vi "test-cubic-spline-02.vi"() -> (3 "Test Passed":bool)   [LabVIEW 2019]
uses:
  <vilib>/Rock Robotics/WPI/ThirdParty/JAS_Junk/TrajLib/POSEwCURVATURE.ctl
  <vilib>/Rock Robotics/WPI/ThirdParty/JAS_Junk/TrajLib/POSE2D.ctl
  <vilib>/Rock Robotics/WPI/ThirdParty/JAS_Junk/TrajLib/TRANSLATION2D.ctl
  <vilib>/Rock Robotics/WPI/ThirdParty/JAS_Junk/TrajLib/ROTATION2D.ctl
  <vilib>/Rock Robotics/WPI/ThirdParty/JAS_Junk/TrajLib/Rotation2d_CreateAngle.vi
  <vilib>/Rock Robotics/WPI/ThirdParty/JAS_Junk/TrajLib/Util_CalcDist.vi
  <vilib>/Rock Robotics/WPI/ThirdParty/JAS_Junk/TrajLib/Trajectory_Library.lvlib
panel:
  out "XY Graph":cluster{dbl[], dbl[]}(graph)
  out "All Interior \nwayPoints\nFound (True)":bool
  out "end rot = 0":dbl
  out "end y = 0":dbl
  out "end x = 0":dbl
  out "start rot = 0":dbl
  out "start y = 0":dbl
  out "start x = 0":dbl
  out "max dtheta < 0.0872":dbl
  out "max dy < 0.00127":dbl
  out "max dx  < 0.127":dbl
  out "Overall Error":errorcluster
  out "Elements":i32
  out "Create Spline Error":errorcluster
  out "SplinePoses\nWCurve":T1[](array[typedef]) {"POSE"."ROTATION"."SIN" format="%13.4f"; "POSE"."ROTATION"."COS" format="%13.4f"; "POSE"."ROTATION"."VALUE" format="%13.4f"; "POSE"."TRANSLATION"."Y" format="%14.3f"; "POSE"."TRANSLATION"."X" format="%14.3f"}
  out "Elapsed Time":dbl
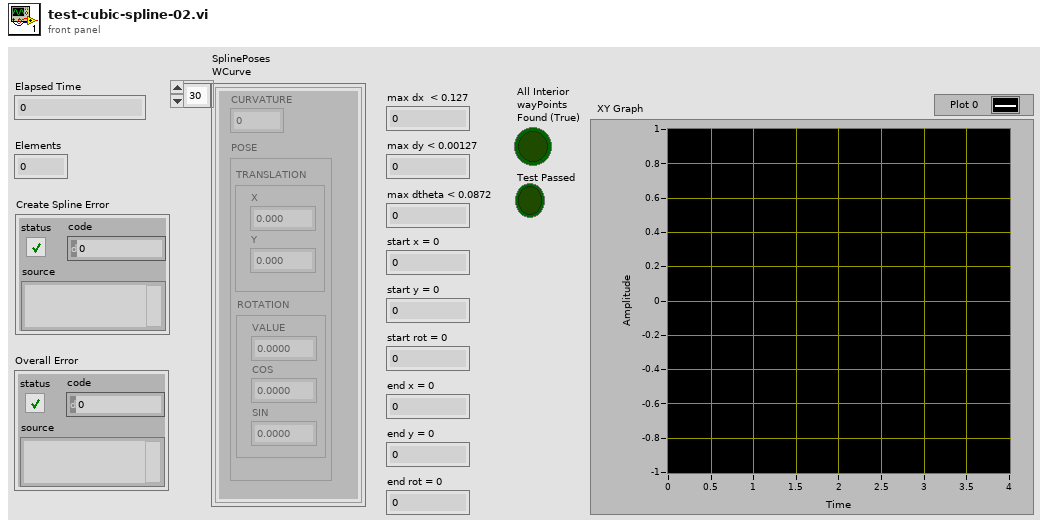
[diagram p1: front panel]
types:
  T1 = typedef "Trajectory_Library.lvlib/POSEwCURVATURE.ctl" = cluster{"CURVATURE":dbl, "POSE":T2}
  T2 = typedef "Trajectory_Library.lvlib/POSE2D.ctl" = cluster{"TRANSLATION":T3, "ROTATION":T4}
  T3 = typedef "Trajectory_Library.lvlib/TRANSLATION2D.ctl" = cluster{"X":dbl, "Y":dbl}
  T4 = typedef "Trajectory_Library.lvlib/ROTATION2D.ctl" = cluster{"VALUE":dbl, "COS":dbl, "SIN":dbl}
  T5 = typedef "Trajectory_Library.lvlib/SPLINE_CTRL_VECTOR.ctl" = cluster{"Xs":dbl[], "Ys":dbl[]}
  T6 = typedef "Trajectory_Library.lvlib/SPLINE.ctl" = cluster{"Degree":i32, "Coefficients":T7}
  T7 = typedef "NI_Matrix.lvlib/RealMatrix.ctl" = dbl[][]
  T8 = typedef "Trajectory_Library.lvlib/TWIST2D.ctl" = cluster{"dX":dbl, "dY":dbl, "dTHETA":dbl}
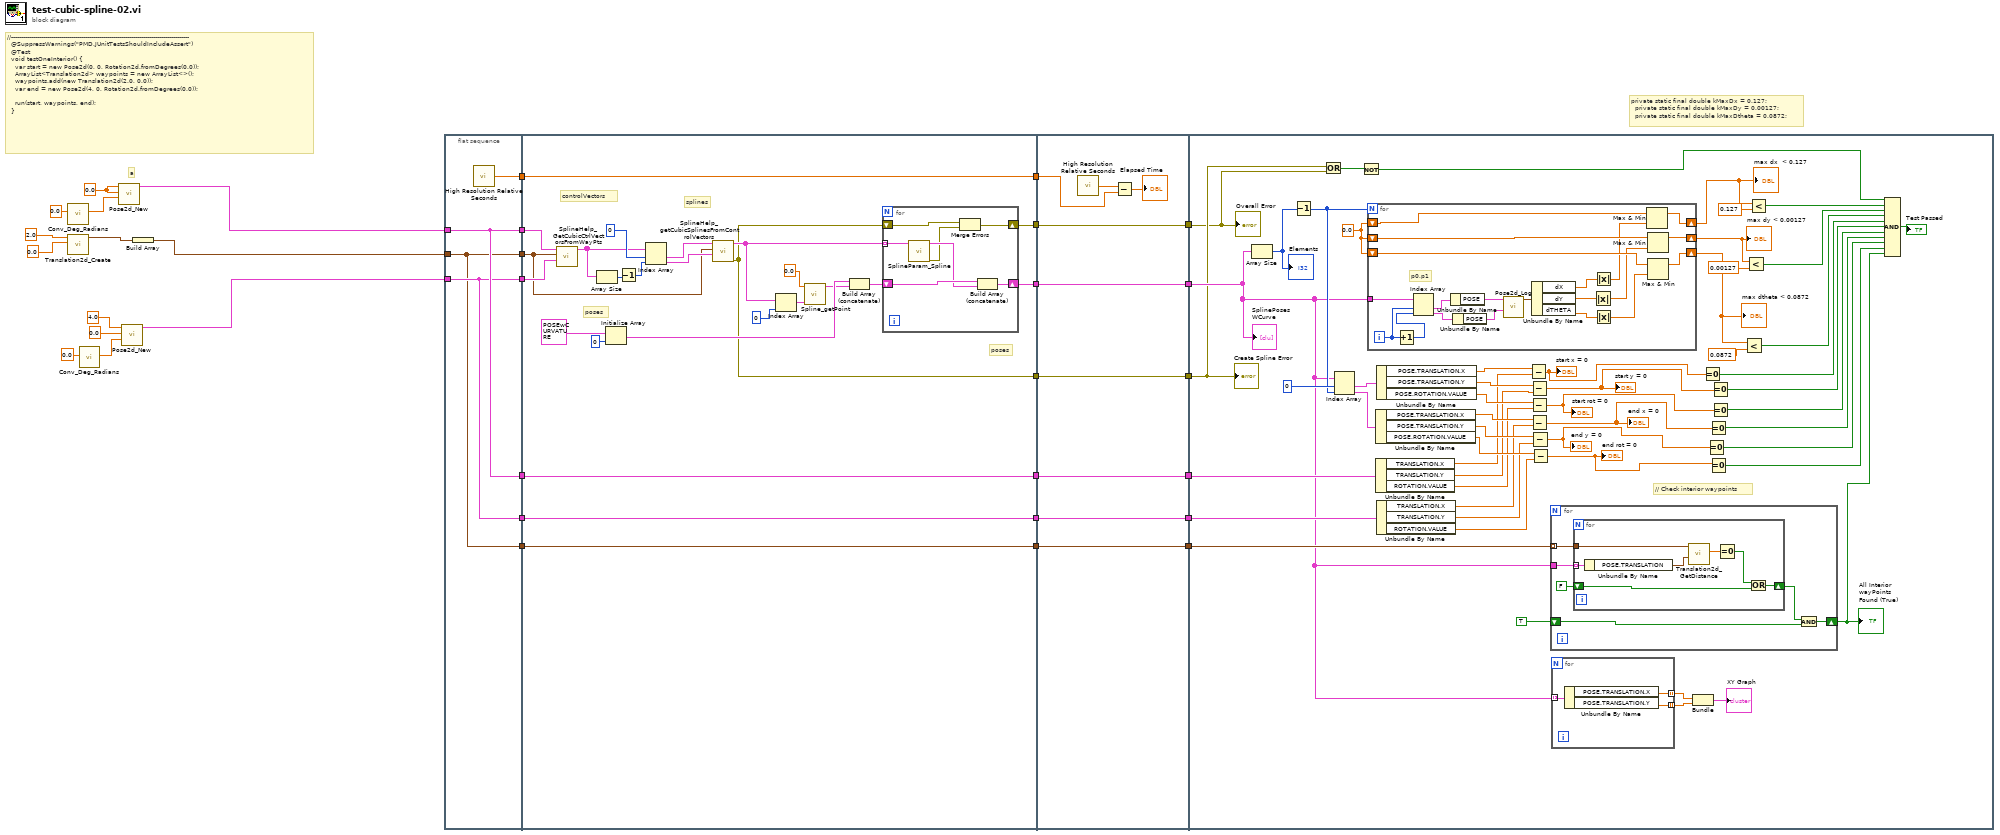
[diagram p0: block diagram]
diagram:
  w11 = 0.0 ("X")
  # "a"
  # "//-----------------------------------------------------------------------------------------\n  @SuppressWarnings(\"PMD.JUnitTestsShouldIncludeAssert\")\n  @Test\n  void testOneInterior() {\n    var start = new Pose2d(0, 0, Rotation2d.fromDegrees(0.0));\n    ArrayList<Translation2d> waypoints = new ArrayList<>();\n    waypoints.add(new Translation2d(2.0, 0.0));\n    var end = new Pose2d(4, 0, Rotation2d.fromDegrees(0.0));\n\n    run(start, waypoints, end);\n  }"
  # "private static final double kMaxDx = 0.127;\n  private static final double kMaxDy = 0.00127;\n  private static final double kMaxDtheta = 0.0872;"
  n1 = call <vilib>:"Conv_Deg_Radians.vi"("Degress"=0.0) -> ("Radians"=w10:dbl)  [unwired: 10 in]
  n2 = call <vilib>:"Translation2d_Create.vi"("Y"=0.0, "X"=2.0) -> ("TRANSLATION"=w8:T3)  [unwired: 9 in]
  n3 = call <vilib>:"Conv_Deg_Radians.vi"("Degress"=0.0) -> ("Radians"=w4:dbl)  [unwired: 10 in]
  n4 = call <vilib>:"Pose2d_New.vi"("Heading"=w10, "Y"=w11, "X"=w11) -> ("out POSe"=w3:T2)  [unwired: 8 in]
  n5 = call <vilib>:"Pose2d_New.vi"("Heading"=w4, "Y"=0.0, "X"=4.0) -> ("out POSe"=w1:T2)  [unwired: 8 in]
  n6 = Build Array(w8) -> (w2:T3[])
  n7 = flat-sequence {
    tunnel: w3 -> [w36]
    tunnel: [w36] -> w33
    tunnel: w2 -> [w34]
    tunnel: [w34] -> w32
    tunnel: w1 -> [w35]
    tunnel: [w35] -> w31
    tunnel: [w37] -> w30
    tunnel: [w36] -> w22
    tunnel: [w35] -> w19
    tunnel: [w34] -> w14
    tunnel: w33 -> [w62]
    tunnel: w32 -> [w54]
    tunnel: w31 -> [w61]
    tunnel: [w53] -> w29
    tunnel: w30 -> [w53]
    tunnel: [w43] -> w28
    tunnel: [w42] -> w26
    tunnel: [w41] -> w24
    tunnel: w22 -> [w40]
    tunnel: [w40] -> w21
    tunnel: w19 -> [w39]
    tunnel: [w39] -> w18
    tunnel: [w38] -> w15
    tunnel: w14 -> [w38]
    tunnel: w29 -> [w78]
    tunnel: w28 -> [w77]
    tunnel: [w77] -> w27
    tunnel: w26 -> [w76]
    tunnel: [w76] -> w25
    tunnel: w24 -> [w75]
    tunnel: [w75] -> w23
    tunnel: w21 -> [w72]
    tunnel: [w72] -> w20
    tunnel: w18 -> [w71]
    tunnel: [w71] -> w17
    tunnel: [w70] -> w16
    tunnel: w15 -> [w70]
    tunnel: w27 -> [w106]
    tunnel: w25 -> [w81]
    tunnel: w23 -> [w80]
    tunnel: w20 -> [w129]
    tunnel: w17 -> [w128]
    tunnel: w16 -> [w111]
    frame #0 {
      n8 = call <vilib>:"High Resolution Relative Seconds.vi"() -> ("relative seconds"=w37:dbl)
    }
    frame #1 {
      # "poses"
      # "poses"
      # "splines"
      # "controlVectors"
      n9 = call <vilib>:"SplineHelp_GetCubicCtrlVectorsFromWayPts.vi"("Enging POSE"=w61, "Interior WAYPOINTS"=w54, "Starting POSE"=w62) -> ("SplineControlVectors"=w58:T5[])  [unwired: 8 in]
      n10 = Array Size(array=w58) -> (size(s)=w59:i32)
      n11 = Initialize Array(T1 {"CURVATURE"=0.0, "POSE"={"TRANSLATION"={"X"=0.0, "Y"=0.0}, "ROTATION"={"VALUE"=0.0, "COS"=1.0, "SIN"=0.0}}} ("POSEwCURVATURE"), 0 ("dimension size")) -> (w47:T1[])
      n12 = Decrement(x=w59) -> (x-1=w57:i32)
      n13 = Index Array(array=w58, index #1=0 ("index"), index #2=w57) -> (element #1=w56:T5, element #2=w55:T5)
      n14 = call <vilib>:"SplineHelp_getCubicSplinesFromControlVectors.vi"("endCtrlVector"=w55, "InternalWaypoints"=w54, "startCtrlVector"=w56) -> ("error out"=w42:errorcluster, "splines"=w44:T6[])  [unwired: 3 in, 4 out]
      n15 = Index Array(array=w44, index=0) -> (element=w49:T6)
      n16 = call <vilib>:"Spline_getPoint.vi"("inputSPLINE"=w49, "Time"=0.0) -> ("POSEwCURVATURE"=w46:T1)  [unwired: 9 in]
      n17 = Build Array (concatenate)(w47, w46) -> (w45:T1[])
      n18 = for {
        shift-right: [w66] -> w43
        shift-left: w45 -> [w68]
        tunnel: w44 -> [w69] mode=indexing
        shift-right: [w64] -> w41
        shift-left: w42 -> [w65]
        n19 = call <vilib>:"SplineParam_Spline.vi"("inputSPLINE"=w69) -> ("error out"=w63:errorcluster, "outputPOSEwCURVATURE"=w67:T1[])  [unwired: 9 in]
        n20 = Merge Errors(w65, w63) -> (w64:errorcluster)
        n21 = Build Array (concatenate)(w68, w67) -> (w66:T1[])
      }
    }
    frame #2 {
      n22 = call <vilib>:"High Resolution Relative Seconds.vi"() -> ("relative seconds"=w73:dbl)
      n23 = Subtract(x=w73, y=w78) -> (x-y=→"Elapsed Time":dbl)
    }
    frame #3 {
      w130 = 0.0
      # "// Check interior waypoints"
      n24 = Array Size(array=w106) -> (size(s)=w131:i32)
      "Elements" <- w131
      n25 = Decrement(x=w131) -> (x-1=w126:i32)
      n26 = Or(x=w81, y=w80) -> (x .or. y?=w82:bool)
      n27 = Index Array(array=w106, index #1=0 ("index"), index #2=w126) -> (element #1=w125:T1, element #2=w124:T1)
      n28 = Not(x=w82) -> (.not. x?=w79:bool)
      n29 = for {
        N: w126 -> [_]
        tunnel: w106 -> [w165]
        shift-right: [w156] -> w103
        shift-left: w130 -> [w153]
        shift-right: [w154] -> w105
        shift-left: w130 -> [w151]
        shift-right: [w155] -> w104
        shift-left: w130 -> [w152]
        i -> [w167]
        # "p0,p1"
        n30 = Increment(x=w167) -> (x+1=w166:i32)
        n31 = Index Array(array=w165, index #1=w167, index #2=w166) -> (element #1=w164:T1, element #2=w163:T1)
        n32 = Unbundle By Name(w164) -> ("POSE"=w162:T2)
        n33 = Unbundle By Name(w163) -> ("POSE"=w161:T2)
        n34 = call <vilib>:"Pose2d_Log.vi"("end POSE"=w161, "in POSE"=w162) -> ("out TWIST"=w160:T8)  [unwired: 9 in]
        n35 = Unbundle By Name(w160) -> ("dX"=w157:dbl, "dY"=w158:dbl, "dTHETA"=w159:dbl)
        n36 = Absolute Value(x=w158) -> (abs(x)=w149:dbl)
        n37 = Absolute Value(x=w157) -> (abs(x)=w150:dbl)
        n38 = Absolute Value(x=w159) -> (abs(x)=w148:dbl)
        n39 = Max & Min(x=w153, y=w150) -> (max(x,y)=w156:dbl)  [unwired: 1 out]
        n40 = Max & Min(x=w152, y=w149) -> (max(x,y)=w155:dbl)  [unwired: 1 out]
        n41 = Max & Min(x=w151, y=w148) -> (max(x,y)=w154:dbl)  [unwired: 1 out]
      }
      "max dx  < 0.127" <- w103
      "max dy < 0.00127" <- w104
      "max dtheta < 0.0872" <- w105
      n42 = Unbundle By Name(w124) -> ("POSE.TRANSLATION.X"=w120:dbl, "POSE.TRANSLATION.Y"=w119:dbl, "POSE.ROTATION.VALUE"=w118:dbl)
      n43 = Unbundle By Name(w129) -> ("TRANSLATION.X"=w117:dbl, "TRANSLATION.Y"=w116:dbl, "ROTATION.VALUE"=w115:dbl)
      n44 = Unbundle By Name(w125) -> ("POSE.TRANSLATION.X"=w123:dbl, "POSE.TRANSLATION.Y"=w122:dbl, "POSE.ROTATION.VALUE"=w121:dbl)
      n45 = Unbundle By Name(w128) -> ("TRANSLATION.X"=w114:dbl, "TRANSLATION.Y"=w113:dbl, "ROTATION.VALUE"=w112:dbl)
      n46 = Subtract(x=w123, y=w117) -> (x-y=w96:dbl)
      "start x = 0" <- w96
      n47 = Subtract(x=w122, y=w116) -> (x-y=w95:dbl)
      "start y = 0" <- w95
      n48 = Subtract(x=w121, y=w115) -> (x-y=w94:dbl)
      "start rot = 0" <- w94
      n49 = Subtract(x=w120, y=w114) -> (x-y=w93:dbl)
      "end x = 0" <- w93
      n50 = Subtract(x=w119, y=w113) -> (x-y=w92:dbl)
      "end y = 0" <- w92
      n51 = Subtract(x=w118, y=w112) -> (x-y=w91:dbl)
      "end rot = 0" <- w91
      n52 = for {
        tunnel: w111 -> [w135] mode=indexing
        tunnel: w106 -> [w140]
        shift-right: [w139] -> w84
        shift-left: TRUE -> [w138]
        n53 = for {
          tunnel: w140 -> [w144] mode=indexing
          shift-right: [w147] -> w136
          shift-left: FALSE -> [w146]
          tunnel: w135 -> [w145]
          n54 = Unbundle By Name(w144) -> ("POSE.TRANSLATION"=w143:T3)
          n55 = call <vilib>:"Translation2d_GetDistance.vi"("other Translation"=w143, "In Translation"=w145) -> ("Distance"=w142:dbl)  [unwired: 9 in]
          n56 = Equal To 0?(x=w142) -> (x = 0?=w141:bool)
          n57 = Or(x=w141, y=w146) -> (x .or. y?=w147:bool)
        }
        n58 = And(x=w136, y=w138) -> (x .and. y?=w139:bool)
      }
      "All Interior \nwayPoints\nFound (True)" <- w84
      n59 = for {
        tunnel: [w134] -> w109 mode=indexing
        tunnel: [w133] -> w108 mode=indexing
        tunnel: w106 -> [w132] mode=indexing
        n60 = Unbundle By Name(w132) -> ("POSE.TRANSLATION.X"=w134:dbl, "POSE.TRANSLATION.Y"=w133:dbl)
      }
      n61 = Bundle(w109, w108) -> (→"XY Graph":cluster{dbl[], dbl[]})  [unwired: 1 in]
      n62 = Equal To 0?(x=w96) -> (x = 0?=w90:bool)
      n63 = Equal To 0?(x=w92) -> (x = 0?=w86:bool)
      n64 = Equal To 0?(x=w93) -> (x = 0?=w87:bool)
      n65 = Equal To 0?(x=w91) -> (x = 0?=w85:bool)
      n66 = Equal To 0?(x=w95) -> (x = 0?=w89:bool)
      n67 = Equal To 0?(x=w94) -> (x = 0?=w88:bool)
      n68 = Less?(x=w105, y=0.0872) -> (x < y?=w97:bool)
      n69 = Less?(x=w104, y=0.00127) -> (x < y?=w98:bool)
      n70 = Less?(x=w103, y=0.127) -> (x < y?=w99:bool)
      n71 = Compound Arithmetic op=AND(w79, w99, w98, w97, w90, w89, w88, w87, w86, w85, w84) -> (→"Test Passed":bool)
      "SplinePoses\nWCurve" <- w106
      "Create Spline Error" <- w81
      "Overall Error" <- w80
    }
  }
